vi "show_chunks.vi"(7 "connection_reference":T2, 8 "error in (no error)":errorcluster, 10 "schema_name":string, 11 "hyper_table_name":string) -> (0 "error out":errorcluster, 3 "chunk []":T1[](array[typedef]) {"start" format="%^<%H:%M:%S%3u %m/%d/%y>T"; "end" format="%^<%H:%M:%S%3u %m/%d/%y>T"})   [LabVIEW 2015, in "lv-timescaledb.lvlib"]
uses:
  lv-timescaledb.lvlib
  <vilib>/addons/database/Connection.llb/Conn ObjectReference.ctl
  _controls/chunk.ctl
  <vilib>/addons/database/Command.llb/Cmd Execute.vi
  <vilib>/addons/database/Recordset.llb/Rec Fetch Recordset Data (CR).vi
  <vilib>/addons/database/Recordset.llb/Rec Destroy - Command.vi
  <vilib>/addons/database/Command.llb/Cmd Delete.vi
  <vilib>/addons/database/NI_Database_API.lvlib
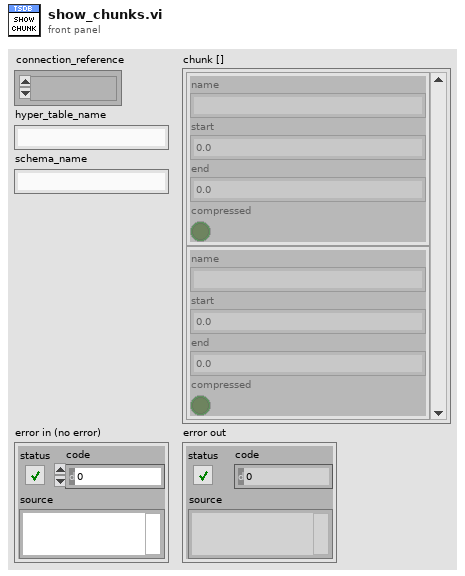
[diagram p1: front panel]
types:
  T1 = typedef "lv-timescaledb.lvlib/chunk.ctl" = cluster{"name":string, "start":dbl, "end":dbl, "compressed":bool}
  T2 = typedef "NI_Database_API.lvlib/Conn ObjectReference.ctl" = refnum<k1>
  T3 = typedef "NI_Database_API.lvlib/DB Tools Parameter Info.ctl" = cluster{"parameter name":string, "type":T4, "direction":T5, "value":variant}
  T4 = typedef "NI_Database_API.lvlib/DB Tools DataTypes.ctl" = enum16{"String", "Long (I32)", "Single (SGL)", "Double (DBL)", "Date/Time", "Binary"}
  T5 = typedef "NI_Database_API.lvlib/DB Tools Parameter Dir.ctl" = enum32{"Input", "Output", "Input/Output", "Return Value"}
  T6 = typedef "NI_Database_API.lvlib/Cmd ObjectReference.ctl" = refnum<k1>
  T7 = typedef "NI_Database_API.lvlib/Cmd-Rec Object Reference.ctl" = refnum<k1>
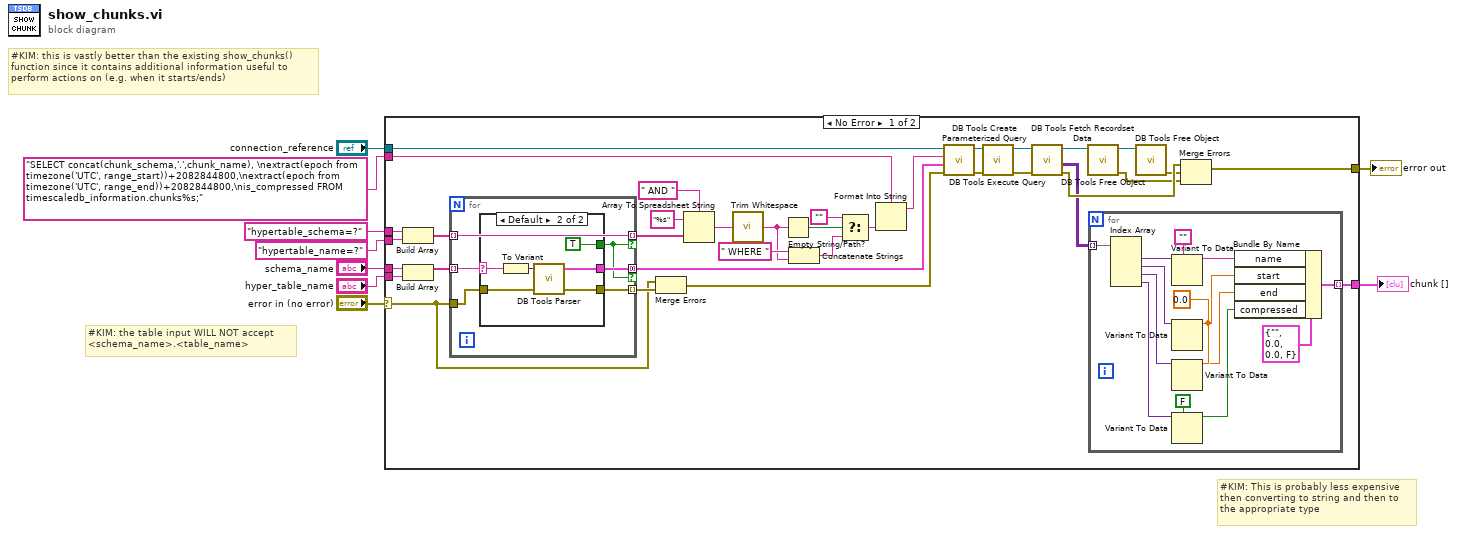
[diagram p0: block diagram]
diagram:
  # "#KIM: the table input WILL NOT accept\n<schema_name>.<table_name>"
  # "#KIM: This is probably less expensive\nthen converting to string and then to\nthe appropriate type"
  # "#KIM: this is vastly better than the existing show_chunks()\nfunction since it contains additional information useful to\nperform actions on (e.g. when it starts/ends)"
  n1 = case shown="No Error" "error in (no error)" {
    selector: "error in (no error)" -> [w15 w72]
    tunnel: "schema_name" -> [w21 _]
    tunnel: "connection_reference" -> [w33 _]
    tunnel: [w43 w72] -> w7
    tunnel: "SELECT concat(chunk_schema,'.',chunk_name), \nextract(epoch from timezone('UTC', range_start))+2082844800,\nextract(epoch from  timezone('UTC', range_end))+2082844800,\nis_compressed FROM timescaledb_information.chunks%s;" -> [w29 _]
    tunnel: "hyper_table_name" -> [w20 _]
    tunnel: [w42 _] -> w3
    tunnel: "hypertable_schema=?" -> [w22 _]
    tunnel: "hypertable_name=?" -> [w19 _]
    frame No Error {
      n2 = Build Array(w22, w19) -> (w17:string[])
      n3 = Build Array(w21, w20) -> (w18:string[])
      n4 = for {
        tunnel: [w49] -> w31 mode=concatenating if=w45
        tunnel: w18 -> [w46] mode=indexing
        tunnel: w15 -> [w50]
        tunnel: [w48] -> w30 mode=indexing
        tunnel: w17 -> [w47] mode=indexing
        tunnel: [w47] -> w14 mode=indexing if=w45
        n5 = case shown="Default" w46 {
          selector: w46 -> [_ w53]
          tunnel: w50 -> [w51 w57]
          tunnel: [_ w55] -> w49
          tunnel: [w51 w54] -> w48
          tunnel: [_ TRUE] -> w45
          frame "" {
          }
          frame Default {
            n6 = To Variant(anything=w53) -> (Variant=w56:variant)
            n7 = call <vilib>:"DB Tools Parser.vi"("error in (no error)"=w57, "variant"=w56) -> ("error out"=w54:errorcluster, "parameters"=w55:T3[])  [unwired: 2 in]
          }
        }
      }
      n8 = Merge Errors(w15, w30) -> (w16:errorcluster)
      n9 = Array To Spreadsheet String(delimiter (Tab)=" AND ", array=w14, 3:"%s" ("format string")) -> (spreadsheet string=w25:string)
      n10 = call <vilib>:"Trim Whitespace.vi"("string"=w25) -> ("trimmed string"=w23:string)  [unwired: 1 in]
      n11 = Empty String/Path?(string/path=w23) -> (empty?=w12:bool)
      n12 = Concatenate Strings(" WHERE ", w23) -> (w11:string)
      n13 = Select(t="", s=w12, f=w11) -> (s? t:f=w13:string)
      n14 = Format Into String(format string=w29, w13) -> (resulting string=w28:string)  [unwired: 2 in, 1 out]
      n15 = call <vilib>:"DB Tools Create Parameterized Query.vi"("error in (no error)"=w16, "parameters"=w31, "SQL query"=w28, "connection reference"=w33) -> ("error out"=w41:errorcluster, "command reference"=w40:T6)  [unwired: 3 in, 1 out]
      n16 = call-poly <vilib>:"DB Tools Execute Query.vi"("error in (no error)"=w41, "command reference"=w40) -> ("error out"=w34:errorcluster, "command-recordset reference"=w37:T7)  [unwired: 6 in]
      n17 = call-poly <vilib>:"DB Tools Fetch Recordset Data.vi"("error in (no error)"=w34, "command-recordset reference"=w37) -> ("error out"=w44:errorcluster, "recordset data"=w32:variant[][], "command-recordset reference out"=w36:T7)  [unwired: 3 in]
      n18 = call-poly <vilib>:"DB Tools Free Object.vi"("command-recordset reference"=w36) -> ("error out"=w38:errorcluster, "command reference"=w35:T6)  [unwired: 9 in]
      n19 = for {
        tunnel: w32 -> [w71] mode=indexing
        tunnel: [w69] -> w42 mode=indexing
        w64 = 0.0
        n20 = Index Array(array=w71) -> (element #1=w68:variant, element #2=w65:variant, element #3=w63:variant, element #4=w59:variant)  [unwired: 4 in]
        n21 = Variant To Data(type="", Variant=w68) -> (data=w67:string)  [unwired: 1 in, 1 out]
        n22 = Variant To Data(type=w64, Variant=w65) -> (data=w62:dbl)  [unwired: 1 in, 1 out]
        n23 = Variant To Data(type=w64, Variant=w63) -> (data=w61:dbl)  [unwired: 1 in, 1 out]
        n24 = Variant To Data(type=FALSE, Variant=w59) -> (data=w60:bool)  [unwired: 1 in, 1 out]
        n25 = Bundle By Name(cluster=T1 {"name"="", "start"=0.0, "end"=0.0, "compressed"=FALSE} ("chunk"), "name"=w67, "start"=w62, "end"=w61, "compressed"=w60) -> (w69:T1)
      }
      n26 = call-poly <vilib>:"DB Tools Free Object.vi"("command reference"=w35) -> ("error out"=w39:errorcluster)  [unwired: 9 in, 1 out]
      n27 = Merge Errors(w44, w39, w38) -> (w43:errorcluster)
    }
    frame Error {
    }
  }
  "error out" <- w7
  "chunk []" <- w3
